vi "Active Word Document Formatted Content.vi"() -> ()   [LabVIEW 2017]
panel:
  out "Formatted String":string
  in  "Word._Application":refnum<k7>
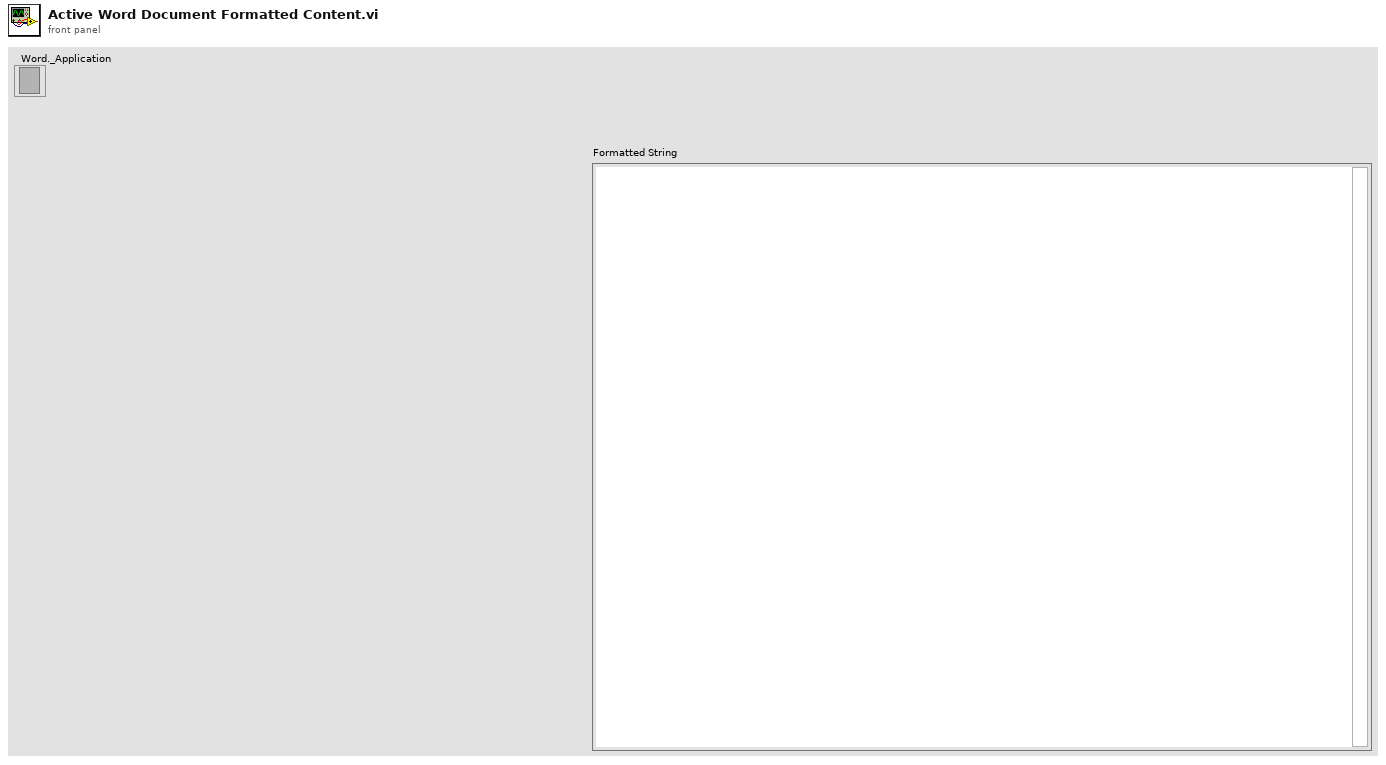
[diagram p1: front panel]
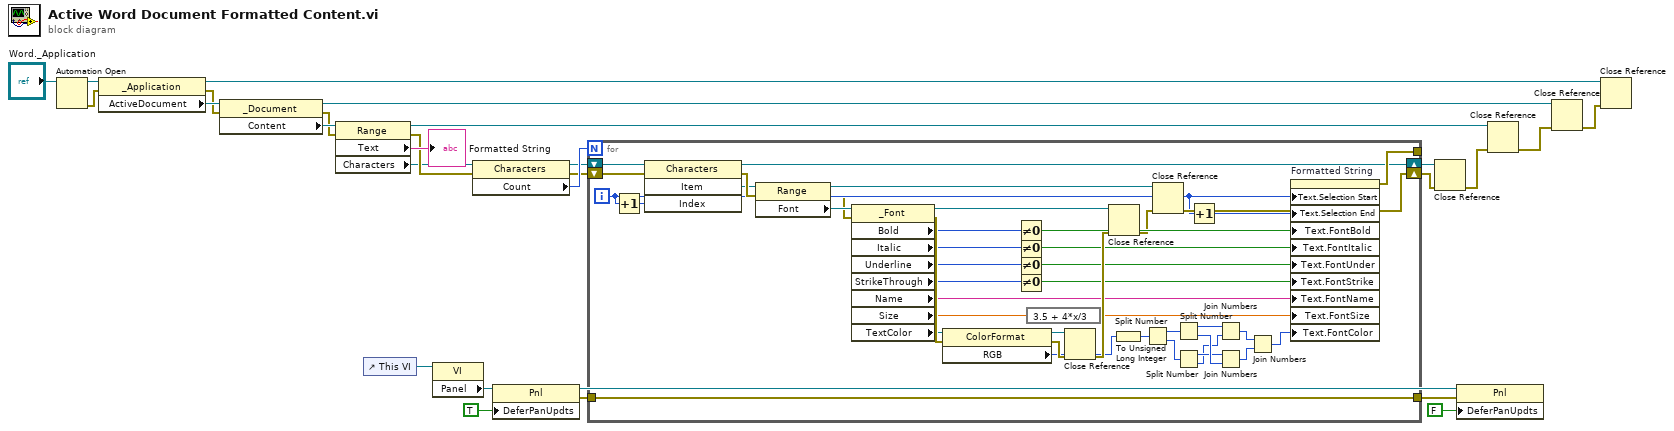
[diagram p0: block diagram]
diagram:
  n1 = Automation Open(Automation Refnum="Word._Application") -> (Automation Refnum=w5:refnum<k7>, error out=w4:errorcluster)  [unwired: 3 in]
  n2 = property class="_Application"(reference=w5, error in=w4) -> (reference out=w7:refnum<k7>, error out=w3:errorcluster, "ActiveDocument"=w28:refnum<k7>)
  n3 = property class="_Document"(reference=w28, error in=w3) -> (reference out=w22:refnum<k7>, error out=w2:errorcluster, "Content"=w27:refnum<k7>)
  n4 = property class="Range"(reference=w27, error in=w2) -> (reference out=w24:refnum<k7>, error out=w9:errorcluster, "Text"=→"Formatted String":string, "Characters"=w1:refnum<k7>)
  n5 = control-ref of="This VI"() -> (w20:refnum<vi>)
  n6 = property class="VI"(reference=w20) -> ("Panel"=w19:refnum<vi>)  [unwired: 1 in, 2 out]
  n7 = property class="Characters"(reference=w1, error in=w9) -> (reference out=w12:refnum<k7>, error out=w13:errorcluster, "Count"=w26:i32)
  n8 = property class="Pnl"(reference=w19, "DeferPanUpdts"=TRUE ("Defer Panel Updates")) -> (reference out=w14:refnum<vi>, error out=w17:errorcluster)  [unwired: 1 in]
  n9 = for {
    N: w26 -> [_]
    shift-right: [w48] -> w25
    shift-left: w12 -> [w71]
    tunnel: w17 -> [w63]
    tunnel: [w63] -> w15
    tunnel: [w62] -> _
    shift-right: [w56] -> w11
    shift-left: w13 -> [w54]
    i -> [w52]
    n10 = Increment(x=w52) -> (x+1=w51:i32)
    n11 = invoke class="Characters" method="Item"(reference=w71, error in=w54, "Index"=w51) -> (reference out=w48:refnum<k7>, error out=w55:errorcluster, "Item"=w53:refnum<k7>)  [unwired: 1 in, 1 out]
    n12 = property class="Range"(reference=w53, error in=w55) -> (reference out=w50:refnum<k7>, error out=w30:errorcluster, "Font"=w70:refnum<k7>)
    n13 = property class="_Font"(reference=w70, error in=w30) -> (reference out=w65:refnum<k7>, error out=w68:errorcluster, "Bold"=w60:i32, "Italic"=w45:i32, "Underline"=w44:i32, "StrikeThrough"=w43:i32, "Name"=w61:string, "Size"=w47:sgl, "TextColor"=w58:refnum<k7>)
    n14 = property class="ColorFormat"(reference=w58, error in=w68) -> (reference out=w67:refnum<k7>, error out=w59:errorcluster, "RGB"=w57:i32)
    n15 = Not Equal To 0?(x=w60) -> (x != 0?=w69:bool)
    n16 = Not Equal To 0?(x=w45) -> (x != 0?=w42:bool)
    n17 = Not Equal To 0?(x=w44) -> (x != 0?=w41:bool)
    n18 = Not Equal To 0?(x=w43) -> (x != 0?=w40:bool)
    n19 = expression code="3.5 + 4*x/3"(w47) -> (w46:sgl)
    n20 = Close Reference(reference=w67, error in (no error)=w59) -> (error out=w66:errorcluster)
    n21 = Close Reference(reference=w65, error in (no error)=w66) -> (error out=w49:errorcluster)
    n22 = To Unsigned Long Integer(number=w57) -> (unsigned 32bit integer=w39:u32)
    n23 = Split Number(x=w39) -> (hi(x)=w38:u16, lo(x)=w37:u16)
    n24 = Close Reference(reference=w50, error in (no error)=w49) -> (error out=w56:errorcluster)
    n25 = Split Number(x=w38) -> (hi(x)=w36:u8, lo(x)=w35:u8)
    n26 = Split Number(x=w37) -> (hi(x)=w34:u8, lo(x)=w29:u8)
    n27 = Increment(x=w52) -> (x+1=w64:i32)
    n28 = Join Numbers(hi=w36, lo=w29) -> ((hi.lo)=w32:u16)
    n29 = Join Numbers(hi=w34, lo=w35) -> ((hi.lo)=w33:u16)
    n30 = Join Numbers(hi=w32, lo=w33) -> ((hi.lo)=w31:u32)
    n31 = property on="Formatted String" class="Str"("Text.Selection Start"=w52, "Text.Selection End"=w64, "Text.FontBold"=w69, "Text.FontItalic"=w42, "Text.FontUnder"=w41, "Text.FontStrike"=w40, "Text.FontName"=w61, "Text.FontSize"=w46, "Text.FontColor"=w31) -> (error out=w62:errorcluster)  [unwired: 2 in, 1 out]
  }
  n32 = Close Reference(reference=w25, error in (no error)=w11) -> (error out=w10:errorcluster)
  n33 = property class="Pnl"(reference=w14, error in=w15, "DeferPanUpdts"=FALSE ("Defer Panel Updates")) -> ()  [unwired: 2 out]
  n34 = Close Reference(reference=w24, error in (no error)=w10) -> (error out=w23:errorcluster)
  n35 = Close Reference(reference=w22, error in (no error)=w23) -> (error out=w8:errorcluster)
  n36 = Close Reference(reference=w7, error in (no error)=w8) -> ()  [unwired: 1 out]
